vi "test-swerve-drive-kinematics-module-state-almost-equal.vi"(4 "Tolerance Deg":dbl=0.1 format="%#_13g", 6 "Tolerance Speed":dbl=0.1 format="%#_13g", 9 "mod State 1":T1={"Speed"=0.0, "Angle"={"VALUE"=0.0, "COS"=1.0, "SIN"=0.0}} {"Angle"."SIN" format="%13.4f"; "Angle"."COS" format="%13.4f"; "Angle"."VALUE" format="%13.4f"}, 11 "mod State 0":T1={"Speed"=0.0, "Angle"={"VALUE"=0.0, "COS"=1.0, "SIN"=0.0}} {"Angle"."SIN" format="%13.4f"; "Angle"."COS" format="%13.4f"; "Angle"."VALUE" format="%13.4f"}) -> (3 "Approx Equal":bool)   [LabVIEW 2019]
uses:
  <vilib>/Rock Robotics/WPI/ThirdParty/JAS_Junk/TrajLib/SWERVE_DRIVE_MODULE_STATE.ctl
  <vilib>/Rock Robotics/WPI/ThirdParty/JAS_Junk/TrajLib/ROTATION2D.ctl
  <vilib>/Rock Robotics/WPI/ThirdParty/JAS_Junk/TrajLib/Trajectory_Library.lvlib
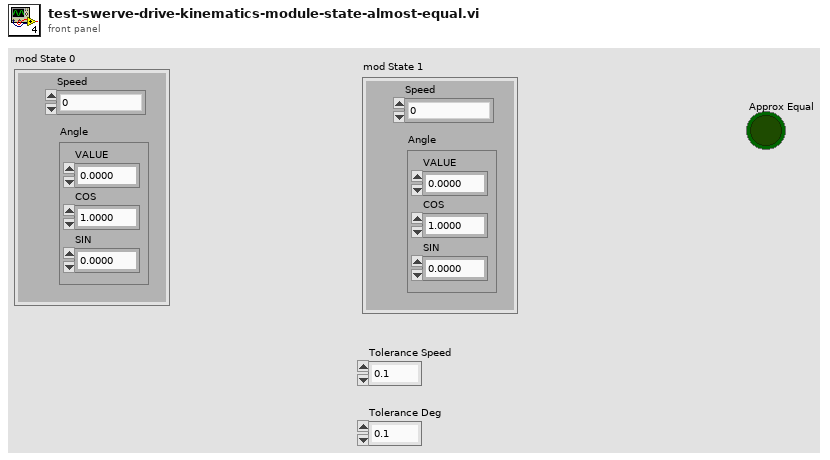
[diagram p1: front panel]
types:
  T1 = typedef "Trajectory_Library.lvlib/SWERVE_DRIVE_MODULE_STATE.ctl" = cluster{"Speed":dbl, "Angle":T2}
  T2 = typedef "Trajectory_Library.lvlib/ROTATION2D.ctl" = cluster{"VALUE":dbl, "COS":dbl, "SIN":dbl}
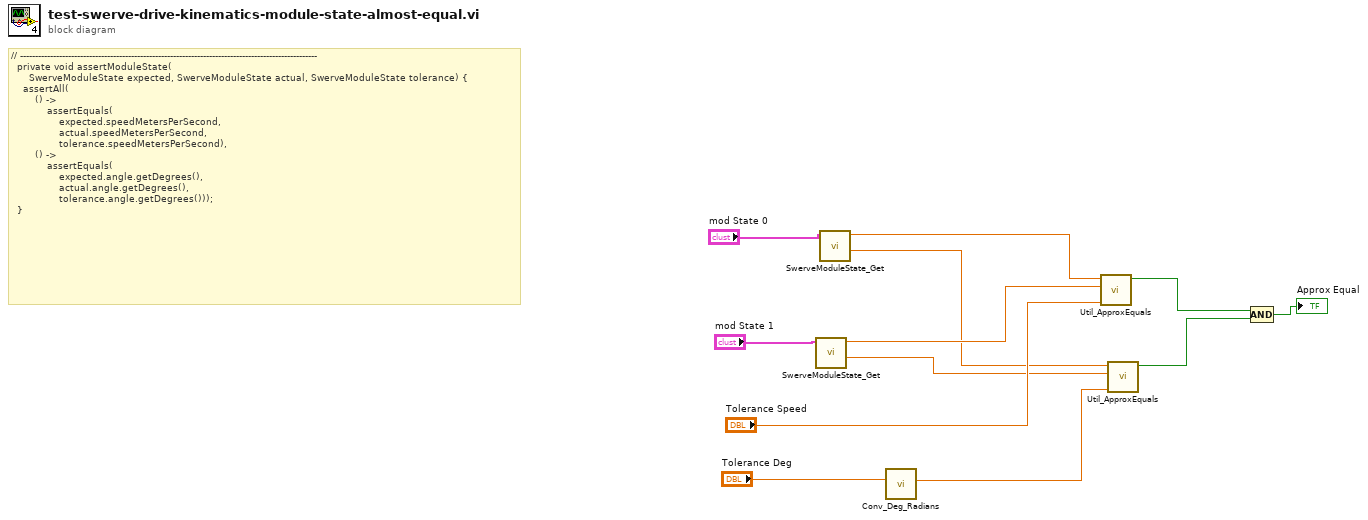
[diagram p0: block diagram]
diagram:
  # "// ---------------------------------------------------------------------------------------------------\n  private void assertModuleState(\n      SwerveModuleState expected, SwerveModuleState actual, SwerveModuleState tolerance) {\n    assertAll(\n        () ->\n            assertEquals(\n                expected.speedMetersPerSecond,\n                actual.speedMetersPerSecond,\n                tolerance.speedMetersPerSecond),\n        () ->\n            assertEquals(\n                expected.angle.getDegrees(),\n                actual.angle.getDegrees(),\n                tolerance.angle.getDegrees()));\n  }"
  n1 = call <vilib>:"SwerveModuleState_Get.vi"("Desired State"="mod State 1") -> ("Angle RADIANS"=w1:dbl, "Speed M/S"=w3:dbl)  [unwired: 9 in]
  n2 = call <vilib>:"SwerveModuleState_Get.vi"("Desired State"="mod State 0") -> ("Angle RADIANS"=w2:dbl, "Speed M/S"=w4:dbl)  [unwired: 9 in]
  n3 = call <vilib>:"Conv_Deg_Radians.vi"("Degress"="Tolerance Deg") -> ("Radians"=w6:dbl)  [unwired: 10 in]
  n4 = call <vilib>:"Util_ApproxEquals.vi"("Tolerance"="Tolerance Speed", "Value 2"=w3, "Value 1"=w4) -> ("ApproxEquals"=w12:bool)  [unwired: 8 in]
  n5 = call <vilib>:"Util_ApproxEquals.vi"("Tolerance"=w6, "Value 2"=w1, "Value 1"=w2) -> ("ApproxEquals"=w11:bool)  [unwired: 8 in]
  n6 = Compound Arithmetic op=AND(w12, w11) -> (→"Approx Equal":bool)
